vi "Get All Objects.vi"(0 "Diagram In":refnum<vi>, 1 "error in":errorcluster) -> (2 "Diagram Out":refnum<vi>, 3 "All Objects":refnum<vi>[](array[refnum]), 4 "error out":errorcluster)   [LabVIEW 2012, in "Scripting Tools.lvlib"]
doc: "Returns all GObjects from the block diagram referenced by <B>Diagram In</B>, including all those in sub-diagrams (loops and sequence structures etc)."
uses:
  Scripting Tools.lvlib
  <vilib>/Utility/traverseref.llb/TRef TravTarget.ctl
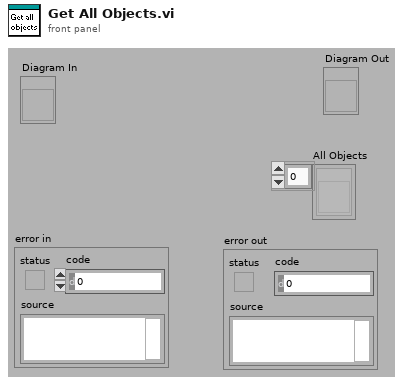
[diagram p1: front panel]
types:
  T1 = typedef "TRef TravTarget.ctl" = enum16{"FP", "BD", "Other"}
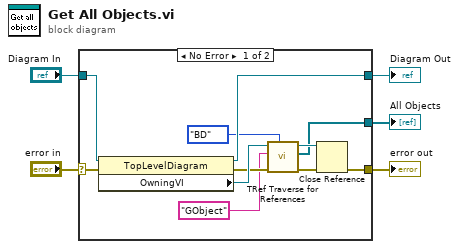
[diagram p0: block diagram]
diagram:
  n1 = case shown="No Error" "error in" {
    selector: "error in" -> [w15 w18]
    tunnel: [w10 w18] -> w5
    tunnel: "Diagram In" -> [w16 w17]
    tunnel: [w9 w17] -> w3
    tunnel: [w8 _] -> w1
    frame No Error {
      n2 = property on="Property Node" class="TopLevelDiagram"(reference=w16, error in=w15) -> (reference out=w9:refnum<vi>, error out=w13:errorcluster, "OwningVI"=w14:refnum<vi>)
      n3 = call <vilib>:"TRef Traverse for References.vi"("Traverse Target"=TRef_TravTarget."BD", "error in (no error)"=w13, "Class Name"="GObject", "VI Refnum"=w14) -> ("error out"=w12:errorcluster, "References"=w8:refnum<vi>[], "dup VI Refnum"=w11:refnum<vi>)  [unwired: 1 in, 4 out]
      n4 = Close Reference(reference=w11, error in (no error)=w12) -> (error out=w10:errorcluster)
    }
    frame Error {
    }
  }
  "error out" <- w5
  "All Objects" <- w1
  "Diagram Out" <- w3
